vi "macro_LinearSystemLoop_SngJntArm_Execute.vi"() -> ()   [LabVIEW 2019, in "Trajectory_Library.lvlib"]
uses:
  Trajectory_Library.lvlib
  Enum/DCMOTOR_TYPES_ENUM.ctl
panel:
  in  "Process Variable\nRadians":dbl
  in  "Ang Pos SP Rad":dbl
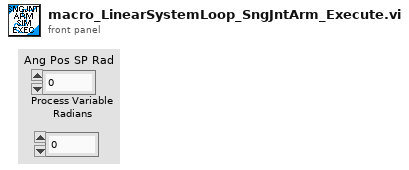
[diagram p1: front panel]
types:
  T1 = typedef "Trajectory_Library.lvlib/DCMOTOR_TYPES_ENUM.ctl" = enum16{"CIM", "AndyMark 9015", "Andy Mark RS 775 125", "Bag", "BaneBots RS 550", "BaneBots RS 775", "Falcon 500", "Mini CIM", "NEO", "NEO 550", "Romi BuiltIn", "Vex 775 Pro", "Snow Blower AM 2235A", "Bosch Seat AM 3493"}
  T2 = typedef "Trajectory_Library.lvlib/LINEAR_SYSTEM_ID_SINGLE_JOINT_ARM_MODEL.ctl" = cluster{"DCMOTOR_TYPES":T1, "Num Motors":i32, "ArmLength_M":dbl, "massKg":dbl, "Gearing":dbl, "MOI kgm2":dbl, "Estimate MOI":bool}
  T3 = typedef "Trajectory_Library.lvlib/LINEAR_SYSTEM_LOOP_SNGJNTARM_CTRL_PARAMS.ctl" = cluster{"Ang Model Std Dev Rad":dbl, "Ang Meas Std Dev Rad":dbl, "Ang Ctrl Tol Rad":dbl, "Max Ctrl Out V":dbl, "Vel Model Std Dev Rad/Sec":dbl, "Vel Ctrl Tol Rad/Sec":dbl}
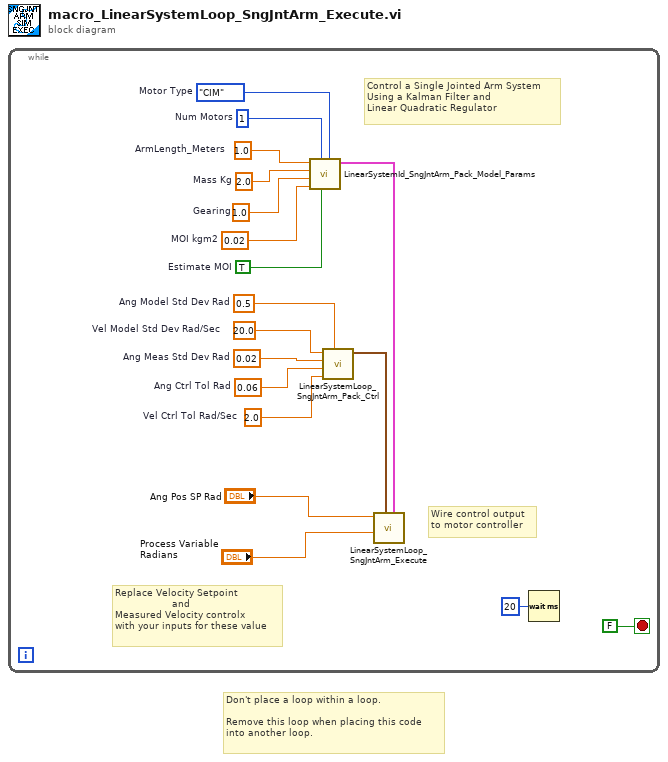
[diagram p0: block diagram]
diagram:
  # "Don't place a loop within a loop.\n \nRemove this loop when placing this code\ninto another loop."
  n1 = while {
    stop <- FALSE stop-if-true
    w1 = 20.0  # Vel Model Std Dev Rad/Sec
    w2 = 0.02  # Ang Meas Std Dev Rad
    w3 = 0.06  # Ang Ctrl Tol Rad
    w4 = 2.0  # Vel Ctrl Tol Rad/Sec
    w5 = 0.5  # Ang Model Std Dev Rad
    w10 = TRUE  # Estimate MOI
    w11 = 0.02  # MOI kgm2
    w12 = 1.0  # ArmLength_Meters
    w15 = 1.0  # Gearing
    w16 = 2.0  # Mass Kg
    w17 = 1  # Num Motors
    w18 = DCMOTOR_TYPES_ENUM."CIM"  # Motor Type
    # "Wire control output\nto motor controller"
    # "Replace Velocity Setpoint \n                   and \nMeasured Velocity controlx\nwith your inputs for these value"
    # "Control a Single Jointed Arm System\nUsing a Kalman Filter and \nLinear Quadratic Regulator"
    n2 = call "LinearSystemId_SngJntArm_Pack_Model_Params.vi"("DCMOTOR_TYPES"=w18, "Estimate MOI"=w10, "Num Motors"=w17, "MOI kgm2"=w11, "Gearing"=w15, "massKg"=w16, "ArmLength_M"=w12) -> ("SngJntArmSim_Model _Params"=w9:T2)  [unwired: 4 in]
    n3 = call "LinearSystemLoop_SngJntArm_Pack_Ctrl.vi"("Ang Model Std Dev Rad"=w5, "Vel Ctrl Tol Rad/Sec"=w4, "Ang Ctrl Tol Rad"=w3, "Ang Meas Std Dev Rad"=w2, "Vel Model Std Dev Rad/Sec"=w1) -> ("LinearSystemLoop_SngJntArm_Ctrl_Params"=w8:T3)  [unwired: 6 in]
    n4 = call "LinearSystemLoop_SngJntArm_Execute.vi"("LinearSystem_ID_SngJntArm_Model"=w9, "LinearSystem_SngJntArm_Ctrl_Params"=w8, "Process Variable\nRadians"="Process Variable\nRadians", "Ang Pos SP Rad"="Ang Pos SP Rad") -> ()  [unwired: 4 in, 4 out]
    n5 = Wait (ms)(milliseconds to wait=u32 20) -> ()  [unwired: 1 out]
  }
